vi "get_sensor_rate.vi"(8 "error in (no error)":errorcluster, 10 "Sensor":u8=1 min=1 max=100 step=1, 11 "VISA resource name":refnum<visa-resource-name>) -> (0 "error out":errorcluster, 2 "Rate (A/s)":dbl, 3 "VISA resource name out":refnum<visa-resource-name>)   [LabVIEW 2018, in "Inficon IC6.lvlib"]
doc: "Query raw sensor rate in A/s. If sensor is not in use response will be 0."
uses:
  <instrlib>/Inficon IC6/Inficon IC6.lvlib
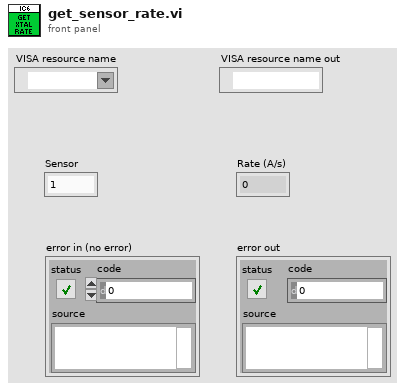
[diagram p1: front panel]
types:
  T1 = enum16{"Source", "General", "Input name", "Process name", "Logic", "Material", "Material name", "Output name", "Process", "Sensor", "Output type", "User message", "Layer", ""}
  T2 = enum16{"Hello", "Query", "Remote action", "Status", "Update"}
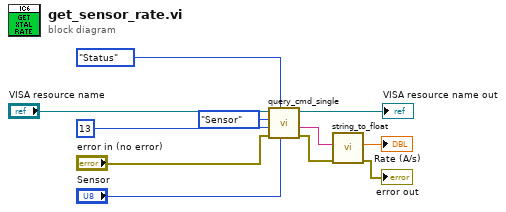
[diagram p0: block diagram]
diagram:
  n1 = call <instrlib>:"query_cmd_single.vi"("Parameter"="Sensor", "Command group"=T2."Status", "error in (no error)"="error in (no error)", "Command ID"=u8 13, "Command subgroup"=T1."Sensor", "VISA resource name"="VISA resource name") -> ("error out"=w3:errorcluster, "formatted response"=w4:string, "VISA resource name out"=→"VISA resource name out":refnum<visa-resource-name>)  [unwired: 1 in, 2 out]
  n2 = call <instrlib>:"string_to_float.vi"("error in (no error)"=w3, "Float (string)"=w4) -> ("error out"=→"error out":errorcluster, "Float (sgl)"=→"Rate (A/s)":sgl)  [unwired: 8 in]
